vi "Roller.vi"(7 "Action":T2, 8 "error in":errorcluster, 10 "RelayValue":T1, 11 "RelayDevRef":T3={"DevStatus"={"status"=FALSE, "code"=0, "source"=""}, "Relay Channel"=enum."Invalid", "Digital Module"=enum."Digital Module 1", "Relay Direction"=enum."Both directions"}) -> (0 "error out":errorcluster)   [LabVIEW 2013]
uses:
  <vilib>/Rock Robotics/WPI/Relay/WPI_RelayDevRef.ctl
  <vilib>/Rock Robotics/SystemInterfaces/DIO/FPGA_DIORelayChannel.ctl
  <vilib>/Rock Robotics/SystemInterfaces/Typedef/FPGA_TypedefDigitalModule.ctl
  <vilib>/Rock Robotics/WPI/Relay/WPI_RelayDirection.ctl
  RollerStates.ctl
  <vilib>/Rock Robotics/WPI/Relay/WPI_RelayValue.ctl
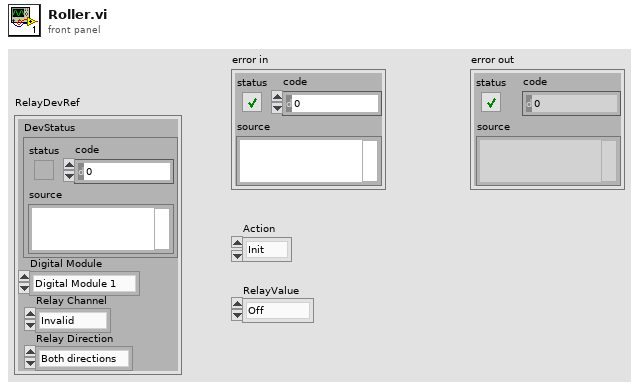
[diagram p1: front panel]
types:
  T1 = typedef "WPI_RelayValue.ctl" = enum16{"Off", "On", "Forward", "Reverse"}
  T2 = typedef "RollerStates.ctl" = enum16{"Init", "SetState", "Disable"}
  T3 = typedef "WPI_RelayDevRef.ctl" = cluster{"DevStatus":errorcluster, "Relay Channel":T4, "Digital Module":T5, "Relay Direction":T6}
  T4 = typedef "FPGA_DIORelayChannel.ctl" = enum8{"Relay 1", "Relay 2", "Relay 3", "Relay 4", "Relay 5", "Relay 6", "Relay 7", "Relay 8", "Invalid"}
  T5 = typedef "FPGA_TypedefDigitalModule.ctl" = enum16{"Digital Module 1", "Digital Module 2"}
  T6 = typedef "WPI_RelayDirection.ctl" = enum16{"Both directions", "Forward only", "Reverse only"}
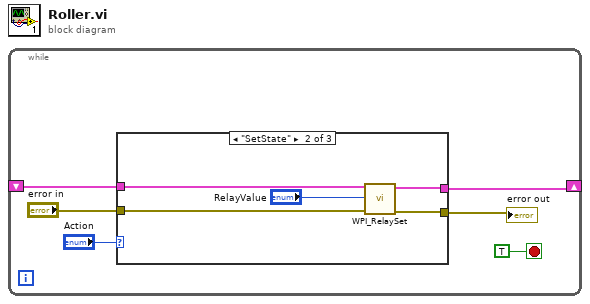
[diagram p0: block diagram]
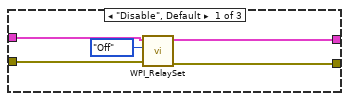
[diagram p2: hidden frame]
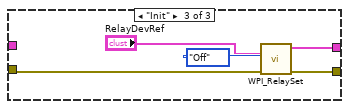
[diagram p3: hidden frame]
diagram:
  n1 = while {
    shift-right: [w4] -> _
    shift-left: _ -> [w5]
    stop <- TRUE stop-if-true
    n2 = case shown="\"SetState\"" "Action" {
      tunnel: w5 -> [w11 w16 _]
      tunnel: [w10 w15 w21] -> w4
      tunnel: [w8 w14 w20] -> w3
      tunnel: "error in" -> [w7 w13 w19]
      frame "Disable", Default {
        n3 = call <vilib>:"WPI_RelaySet.vi"("error in (no error)"=w7, "RelayValue"=WPI_RelayValue."Off", "RelayDevRef"=w11) -> ("error out"=w8:errorcluster, "RelayDevRef"=w10:T3)  [unwired: 7 in]
      }
      frame "SetState" {
        n4 = call <vilib>:"WPI_RelaySet.vi"("error in (no error)"=w13, "RelayValue"="RelayValue", "RelayDevRef"=w16) -> ("error out"=w14:errorcluster, "RelayDevRef"=w15:T3)  [unwired: 7 in]
      }
      frame "Init" {
        n5 = call <vilib>:"WPI_RelaySet.vi"("error in (no error)"=w19, "RelayValue"=WPI_RelayValue."Off", "RelayDevRef"="RelayDevRef") -> ("error out"=w20:errorcluster, "RelayDevRef"=w21:T3)  [unwired: 7 in]
      }
    }
    "error out" <- w3
  }
